vi "Function.vi"(8 "error in (no error)":errorcluster, 9 "Numeric B":u64, 10 "Numeric A":u64, 11 "Two Terminal in":refnum<class "Equal_U64.lvclass">) -> (0 "error out":errorcluster, 2 "Result":bool, 3 "Two Terminal out":refnum<class "Equal_U64.lvclass">)   [LabVIEW 2021, in "Equal_U64.lvclass"]
uses:
  Equal_U64.lvclass
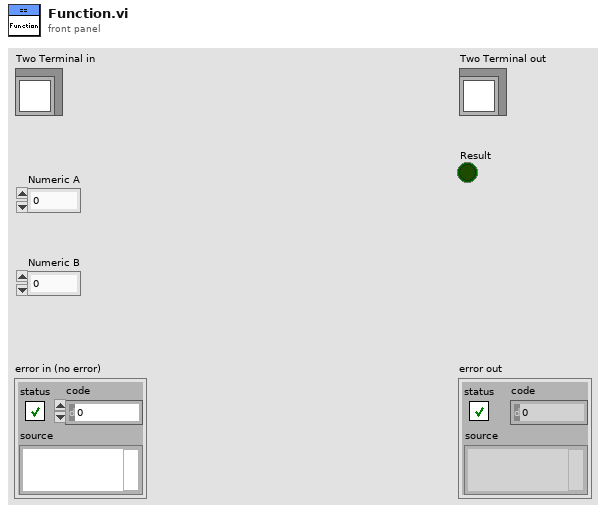
[diagram p1: front panel]
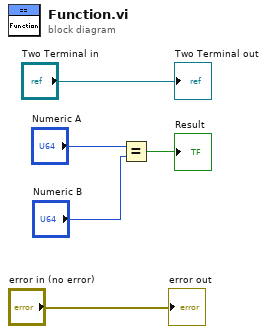
[diagram p0: block diagram]
diagram:
  n1 = Equal?(x="Numeric A", y="Numeric B") -> (x = y?=→"Result":bool)
  "error out" <- "error in (no error)"
  "Two Terminal out" <- "Two Terminal in"
